vi "Write Data.vi"(8 "error in (no error)":errorcluster, 10 "Data":refnum<class "Data.lvclass">[](array[class]), 11 "UI Actor in":refnum<class "UI Actor.lvclass">) -> (0 "error out":errorcluster, 3 "UI Actor out":refnum<class "UI Actor.lvclass">)   [LabVIEW 2014, in "Device Test.lvlib" / "UI Actor.lvclass"]
uses:
  UI Actor.lvclass
  reusable/Data/Data.lvclass
  UI Actor.lvclass/UI Actor.ctl
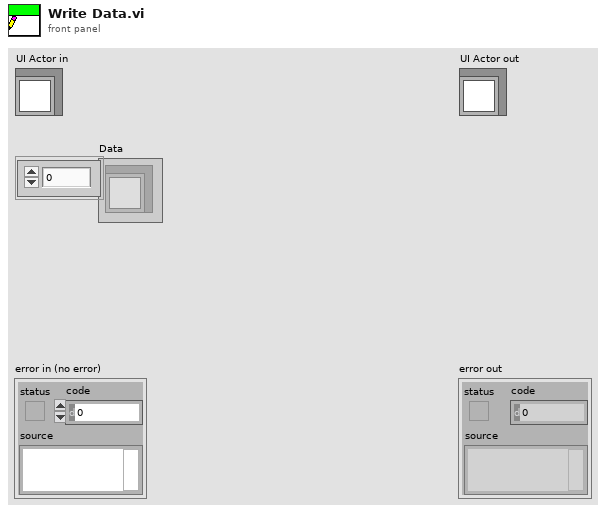
[diagram p1: front panel]
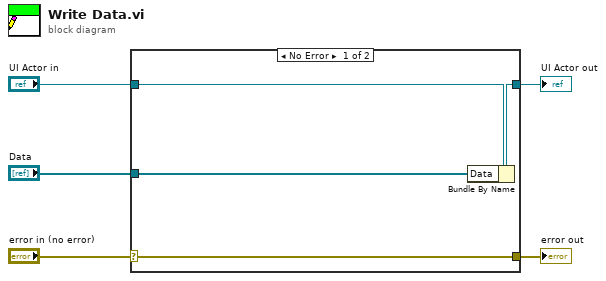
[diagram p0: block diagram]
diagram:
  n1 = case shown="No Error" "error in (no error)" {
    selector: "error in (no error)" -> [w9 w10]
    tunnel: [w9 w10] -> w4
    tunnel: [w7 w11] -> w2
    tunnel: "UI Actor in" -> [w8 w11]
    tunnel: "Data" -> [w6 _]
    frame No Error {
      n2 = Bundle By Name(cluster=w8, "Data"=w6) -> (w7:refnum<class "UI Actor.lvclass">)
    }
    frame Error {
    }
  }
  "error out" <- w4
  "UI Actor out" <- w2
